vi "Idler.vi"(8 "Mission Array In":refnum<class "GenericMission.lvclass">[](array[class]), 9 "BoatLocation":refnum<notifier>, 11 "currently idling?":bool=TRUE) -> (0 "Mission Array out":refnum<class "GenericMission.lvclass">[](array[class]), 3 "still idling?":bool=TRUE)   [LabVIEW 2013]
doc: "Detects when the boat should be in idle mode and implements an idle mission.\n\nKaitlin 4/23"
uses:
  Classes/Missions/GenericMission/GenericMission.lvclass
  Data/TypeDefs/UTM Location.ctl
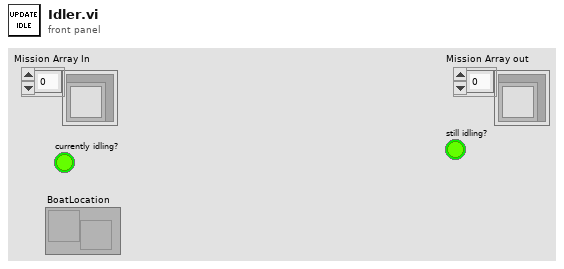
[diagram p1: front panel]
types:
  T1 = typedef "UTM Location.ctl" = cluster{"UTM Zone":dbl, "Hemisphere":enum16{"North", "South"}, "East":dbl, "North":dbl}
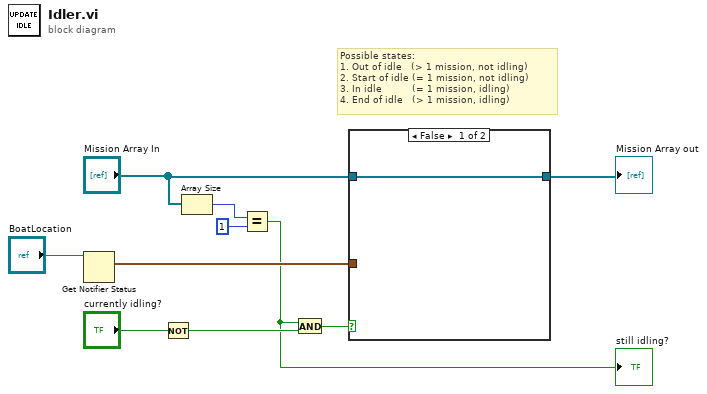
[diagram p0: block diagram]
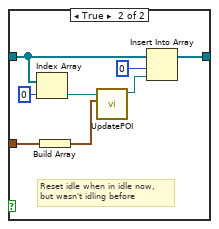
[diagram p2: hidden frame]
diagram:
  # "Possible states:\n1. Out of idle   (> 1 mission, not idling)\n2. Start of idle (= 1 mission, not idling)\n3. In idle          (= 1 mission, idling)\n4. End of idle   (> 1 mission, idling)"
  n1 = Get Notifier Status(notifier="BoatLocation") -> (current notification=w5:T1)  [unwired: 1 in, 4 out]
  n2 = Not(x="currently idling?") -> (.not. x?=w2:bool)
  n3 = Array Size(array="Mission Array In") -> (size(s)=w10:i32)
  n4 = Equal?(x=w10, y=1) -> (x = y?=w1:bool)
  "still idling?" <- w1
  n5 = And(x=w1, y=w2) -> (x .and. y?=w3:bool)
  n6 = case shown="False" w3 {
    tunnel: "Mission Array In" -> [w11 w17]
    tunnel: [w11 w18] -> w7
    tunnel: w5 -> [_ w12]
    frame False {
    }
    frame True {
      # "Reset idle when in idle now,\nbut wasn't idling before"
      n7 = Index Array(array=w17, index=0) -> (element=w14:refnum<class "GenericMission.lvclass">)
      n8 = Build Array(w12) -> (w13:T1[])
      n9 = call-dynamic "UpdatePOI.vi"("Points of Interest"=w13, "GenericMission in"=w14) -> ("GenericMission out"=w16:refnum<class "GenericMission.lvclass">)  [unwired: 8 in, 1 out]
      n10 = Insert Into Array(array=w17, index=0, new element=w16) -> (w18:refnum<class "GenericMission.lvclass">[])
    }
  }
  "Mission Array out" <- w7
